vi "Send Configure Fixed Ref Junction [TC].vi"(7 "Message Priority (Normal)":T1=enum."Normal", 8 "error in (no error)":errorcluster, 10 "fixed ref junc (0.0 Celsius)":dbl format="%^.2e", 11 "Message Enqueuer":refnum<class "Message Enqueuer.lvclass">) -> (0 "error out":errorcluster, 3 "Message Enqueuer out":refnum<class "Message Enqueuer.lvclass">)   [LabVIEW 2015, in "CS++DMM.lvlib" / "Configure Fixed Ref Junction [TC] Msg.lvclass"]
doc: "Sends the <B>CS++DMM.lvlib:Configure Fixed Ref Junction [TC] Msg.lvclass</B> message.\n\n<B>CS++DMM.lvlib:CS++DMM.lvclass:Configure Fixed Ref Junction [TC].vi</B> Description:\n\nThis VI configures the fixed reference junction for a thermocouple with a fixed reference junction type.\n\nThis VI affects the behavior of the instrument only when the IviDmm>Temperature Measurements>Thermocouple>Reference Junction Type [TC] property is set to IVIDMM_VAL_TEMP_REF_JUNC_FIXED.\n\nNote:\n\n(1) This VI is part of the IviDmmThermocouple [TC] extension group."
uses:
  Configure Fixed Ref Junction [TC] Msg.lvclass
  <vilib>/ActorFramework/Message Enqueuer/Message Enqueuer.lvclass
  <vilib>/ActorFramework/Message Enqueuer/Message Priority.ctl
  Configure Fixed Ref Junction [TC] Msg.lvclass/Configure Fixed Ref Junction [TC] Msg.ctl
  <vilib>/ActorFramework/Message Enqueuer/Message Enqueuer.lvclass/Message Enqueuer.ctl
  <vilib>/ActorFramework/Message Priority Queue/Priority Enqueue.vi
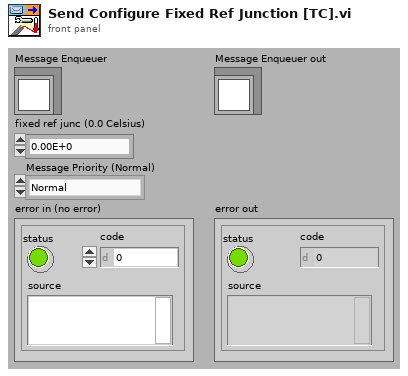
[diagram p1: front panel]
types:
  T1 = typedef "Actor Framework.lvlib/Message Enqueuer.lvclass/Message Priority.ctl" = enum16{"Low", "Normal", "High"}
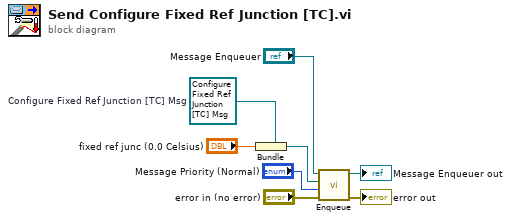
[diagram p0: block diagram]
diagram:
  w2 = refnum<class "Configure Fixed Ref Junction [TC] Msg.lvclass"> refnum  # Configure Fixed Ref Junction [TC] Msg
  n1 = Bundle(cluster=w2, "fixed ref junc (0.0 Celsius)") -> (w5:refnum<class "Configure Fixed Ref Junction [TC] Msg.lvclass">)
  n2 = call <vilib>:"Enqueue.vi"("error in (no error)"="error in (no error)", "Message Priority (Normal)"="Message Priority (Normal)", "Message"=w5, "Message Enqueuer in"="Message Enqueuer") -> ("error out"=→"error out":errorcluster, "Message Enqueuer out"=→"Message Enqueuer out":refnum<class "Message Enqueuer.lvclass">)  [unwired: 6 in]
